vi "Send period commands.vi"(5 "Reading type ref":refnum<vi>, 7 "Fs ref":refnum<vi>, 11 "data value reference":refnum<data-value>) -> ()   [LabVIEW 2017]
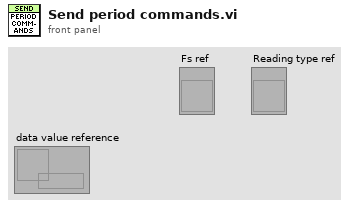
[diagram p1: front panel]
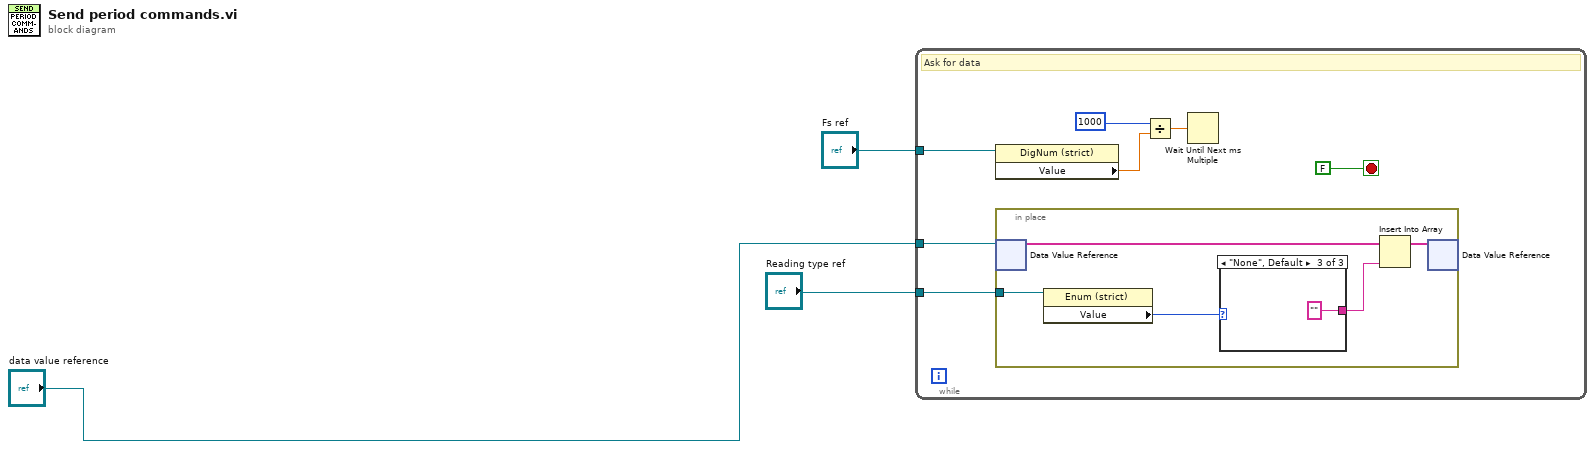
[diagram p0: block diagram]
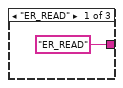
[diagram p2: hidden frame]
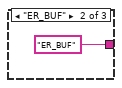
[diagram p3: hidden frame]
diagram:
  n1 = while {
    tunnel: "data value reference" -> [w9]
    tunnel: "Fs ref" -> [w6]
    tunnel: "Reading type ref" -> [w4]
    stop <- FALSE stop-if-true
    # "Ask for data"
    n2 = property class="DigNum (strict)"(reference=w6) -> ("Value"=w5:dbl)  [unwired: 1 in, 2 out]
    n3 = in-place {
      in-place-border: w4 -> [w12]
      n4 = in-place-dvr #1(w9) -> (w15:string[])  [unwired: 1 out]
      n5 = property class="Enum (strict)"(reference=w12) -> ("Value"=w11:enum16{"ER_READ", "ER_BUF", "None"})  [unwired: 1 in, 2 out]
      n6 = case shown="\"None\", Default" w11 {
        tunnel: ["ER_READ" ("new element/subarray") "ER_BUF" ("new element/subarray") "" ("new element/subarray")] -> w13
        frame "ER_READ" {
        }
        frame "ER_BUF" {
        }
        frame "None", Default {
        }
      }
      n7 = Insert Into Array(array=w15, new element=w13) -> (w14:string[])  [unwired: 1 in]
      n8 = in-place-dvr #1(w14) -> ()  [unwired: 2 out]
    }
    n9 = Divide(x=1000, y=w5) -> (x/y=w8:dbl)
    n10 = Wait Until Next ms Multiple(millisecond multiple=w8) -> ()  [unwired: 1 out]
  }
